vi "Double Page.vi"(8 "error in (no error)":errorcluster, 11 "Node Ptr":T1 format="%.0x") -> (0 "error out":errorcluster)   [LabVIEW 2012, in "Shared Variable Custom Device.lvlib"]
uses:
  Shared Variable Custom Device.lvlib
  <vilib>/NI Veristand/Custom Device API/Custom Device Item Ref.ctl
  <vilib>/NI Veristand/Custom Device API/Custom Device API.lvlib
panel:
  in  "Units":string
  out "Network-Published Shared Variable URL":string
  in  "Header":cluster{"Section Name":string}={"Section Name"="Custom Device Item Settings"}
  in  "Description":string
  in  "Name":string
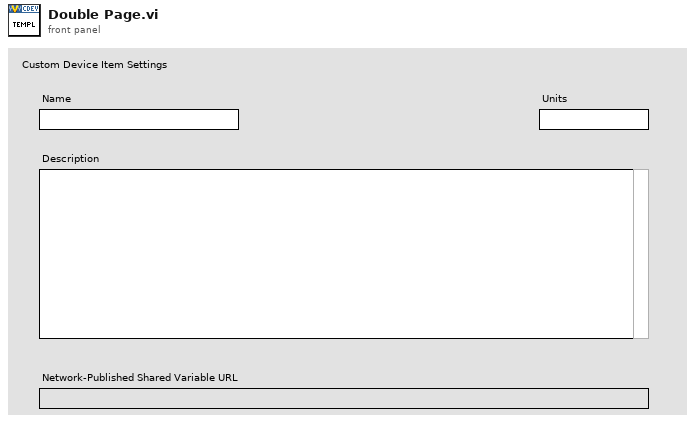
[diagram p1: front panel]
types:
  T1 = typedef "Custom Device API.lvlib/Custom Device Item Ref.ctl" = u64
  T2 = typedef "Custom Device API.lvlib/Custom Device Item Info.ctl" = cluster{"Name":string, "Is Channel":bool, "GUID":string, "Is Waveform":bool}
  T3 = typedef "Custom Device API.lvlib/Custom Device Channel.ctl" = cluster{"Type":T4, "Units":string, "Default Value":dbl, "Faultable":bool, "Scalable":bool}
  T4 = typedef "Custom Device API.lvlib/Custom Device Channel Type.ctl" = enum16{"Input", "Output"}
  T5 = typedef "Custom Device API.lvlib/Custom Device Commands.ctl" = enum16{"Default", "Item renamed", "Shutdown", "Dynamic button pressed"}
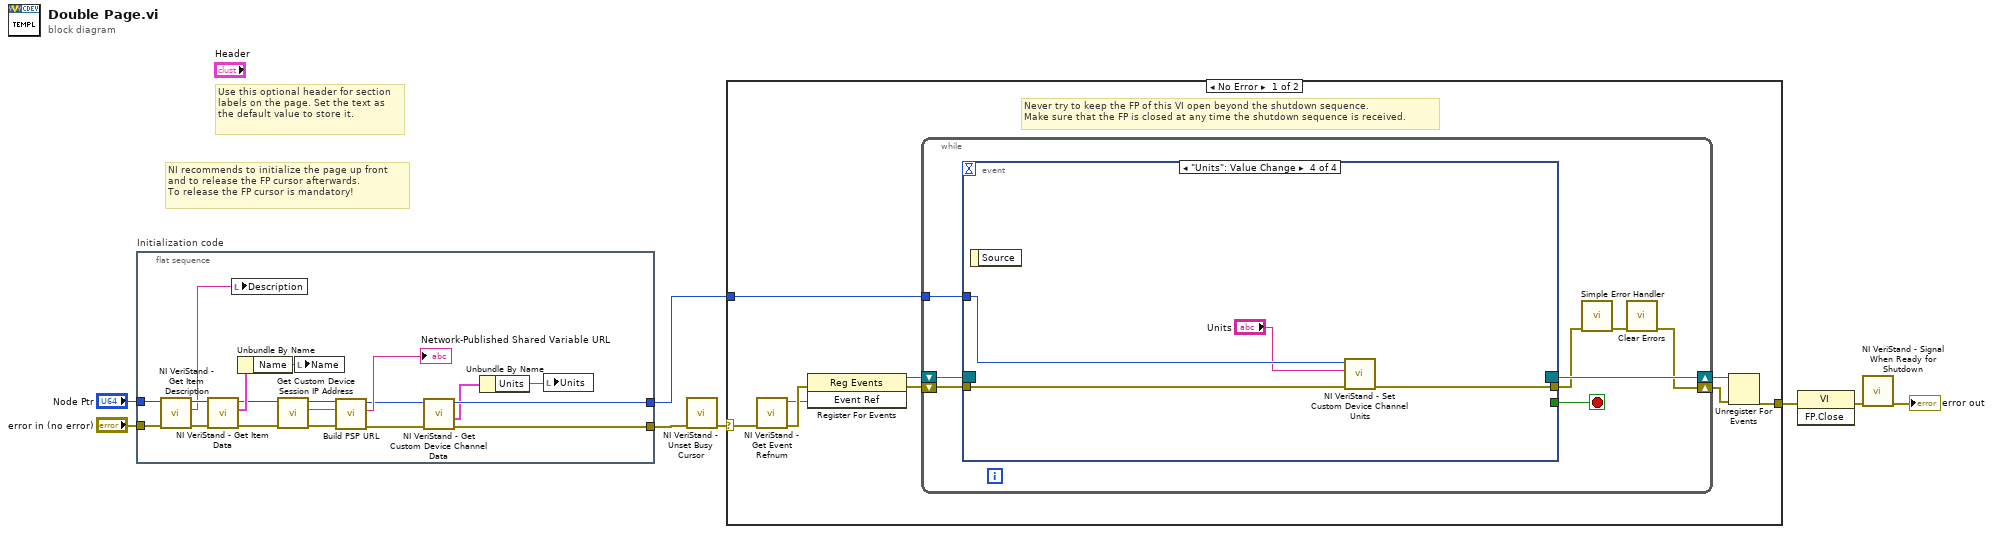
[diagram p0: block diagram]
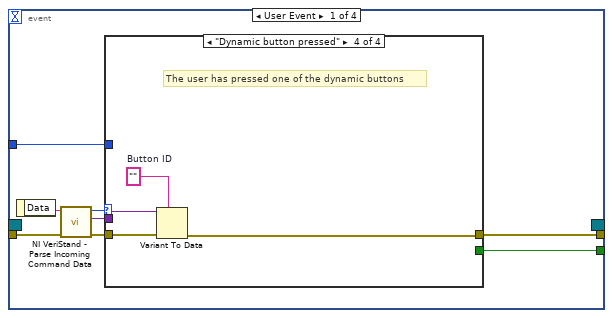
[diagram p2: hidden frame]
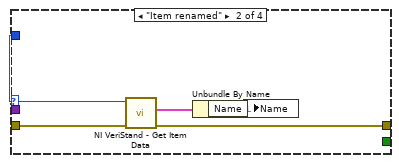
[diagram p4: hidden frame]
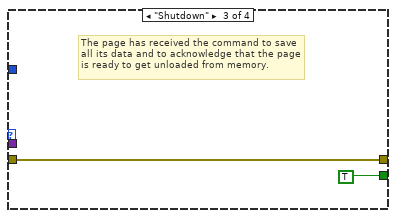
[diagram p5: hidden frame]
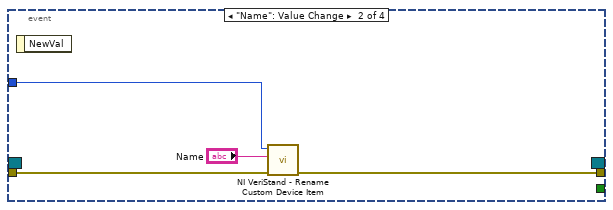
[diagram p6: hidden frame]
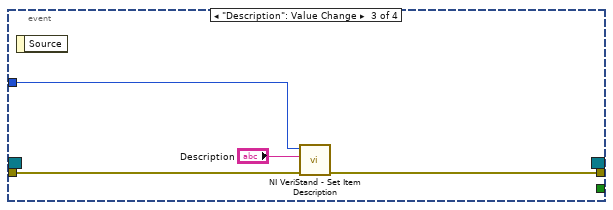
[diagram p7: hidden frame]
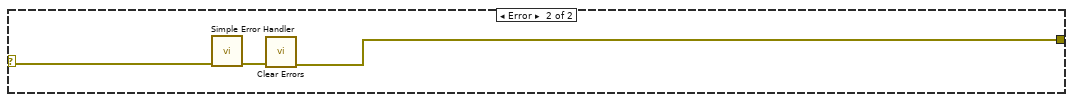
[diagram p8: hidden frame]
diagram:
  # "Use this optional header for section labels on the page. Set the text as the default value to store it."
  # "NI recommends to initialize the page up front\nand to release the FP cursor afterwards.\nTo release the FP cursor is mandatory!"
  n1 = flat-sequence "Initialization code" {
    tunnel: "error in (no error)" -> [w26]
    tunnel: "Node Ptr" -> [w25]
    tunnel: [w11] -> w4
    tunnel: [w12] -> w1
    frame #0 {
      n2 = call <vilib>:"NI VeriStand - Get Item Description.vi"("error in (no error)"=w26, "Item Ref in"=w25) -> ("error out"=w23:errorcluster, "Description"=w24:string, "Item Ref out"=w27:T1)  [unwired: 7 out]
      n3 = call <vilib>:"NI VeriStand - Get Item Data.vi"("error in (no error)"=w23, "Item Ref in"=w27) -> ("error out"=w19:errorcluster, "Item Info"=w22:T2, "Item Ref out"=w20:T1)  [unwired: 7 out]
      n4 = local write "Description"(w24) -> ()
      n5 = Unbundle By Name(w22) -> ("Name"=w21:string)
      n6 = call "Get Custom Device Session IP Address.vi"("error in (no error)"=w19, "Item Ref in"=w20) -> ("error out"=w16:errorcluster, "IP Address"=w17:string, "Item Ref out"=w18:T1)  [unwired: 7 in]
      n7 = local write "Name"(w21) -> ()
      n8 = call "Build PSP URL.vi"("error in (no error)"=w16, "IP Address"=w17, "Channel Ref in"=w18) -> ("error out"=w13:errorcluster, "Shared Variable URL"=→"Network-Published Shared Variable URL":string, "Channel Ref out"=w14:T1)  [unwired: 6 in]
      n9 = call <vilib>:"NI VeriStand - Get Custom Device Channel Data.vi"("error in (no error)"=w13, "Channel Ref in"=w14) -> ("error out"=w11:errorcluster, "Channel"=w10:T3, "Channel Ref out"=w12:T1)  [unwired: 4 in, 3 out]
      n10 = Unbundle By Name(w10) -> ("Units"=w9:string)
      n11 = local write "Units"(w9) -> ()
    }
  }
  n12 = call <vilib>:"NI VeriStand - Unset Busy Cursor.vi"("error in (no error)"=w4) -> ("error out"=w3:errorcluster)  [unwired: 10 out]
  n13 = case shown="No Error" w3 {
    selector: w3 -> [w28 w79]
    tunnel: [w33 w77] -> w8
    tunnel: w1 -> [w29 _]
    frame No Error {
      # "Never try to keep the FP of this VI open beyond the shutdown sequence.\nMake sure that the FP is closed at any time the shutdown sequence is received."
      n14 = call <vilib>:"NI VeriStand - Get Event Refnum.vi"("error in (no error)"=w28) -> ("error out"=w36:errorcluster, "Event Ref"=w32:refnum<user-event>)  [unwired: 9 out]
      n15 = register-events(error in=w36, w32) -> (reference out=w30:refnum<event-registration>, error out=w31:errorcluster)  [unwired: 1 in]
      n16 = while {
        tunnel: w29 -> [w40]
        shift-right: [w37] -> w34
        shift-left: w31 -> [w43]
        shift-right: [w44] -> w35
        shift-left: w30 -> [w42]
        stop <- w41 stop-if-true
        n17 = event shown="[3] \"Units\": Value Change" {
          selector: w42 -> [_ _ _ _]
          dyn-events: [_ _ _ _] -> w44
          timeout: _ -> [_ _ _ _]
          tunnel: w43 -> [w52 w68 w71 w75]
          tunnel: [w48 _ _ _] -> w41
          tunnel: [w47 w67 w70 w73] -> w39
          tunnel: w40 -> [w46 w66 w72 w76]
          event User Event {
            n18 = event-data() -> ("Data"=w51:string)  [unwired: 1 out]
            n19 = call <vilib>:"NI VeriStand - Parse Incoming Command Data.vi"("error in (no error)"=w52, "Incoming data"=w51) -> ("error out"=w50:errorcluster, "Outgoing data"=w45:variant, "Action"=w49:T5)  [unwired: 7 out]
            n20 = case shown="\"Dynamic button pressed\"" w49 {
              tunnel: w50 -> [w53 w58 w59 w64]
              tunnel: [_ _ TRUE _] -> w48
              tunnel: [w53 w55 w59 w61] -> w47
              tunnel: w46 -> [_ w57 _ _]
              tunnel: w45 -> [_ _ _ w63]
              frame "Default", Default {
              }
              frame "Item renamed" {
                n21 = call <vilib>:"NI VeriStand - Get Item Data.vi"("error in (no error)"=w58, "Item Ref in"=w57) -> ("error out"=w55:errorcluster, "Item Info"=w56:T2)  [unwired: 8 out]
                n22 = Unbundle By Name(w56) -> ("Name"=w54:string)
                n23 = local write "Name"(w54) -> ()
              }
              frame "Shutdown" {
                # "The page has received the command to save all its data and to acknowledge that the page is ready to get unloaded from memory."
              }
              frame "Dynamic button pressed" {
                w62 = ""  # Button ID
                # "The user has pressed one of the dynamic buttons"
                n24 = Variant To Data(error in=w64, type=w62, Variant=w63) -> (error out=w61:errorcluster)  [unwired: 1 out]
              }
            }
          }
          event "Name": Value Change {
            n25 = event-data() -> ()  [unwired: 2 out]
            n26 = call <vilib>:"NI VeriStand - Rename Custom Device Item.vi"("error in (no error)"=w68, "New Name"="Name", "Item Ref in"=w66) -> ("error out"=w67:errorcluster)  [unwired: 1 in, 7 out]
          }
          event "Description": Value Change {
            n27 = event-data() -> ()  [unwired: 2 out]
            n28 = call <vilib>:"NI VeriStand - Set Item Description.vi"("error in (no error)"=w71, "Description"="Description", "Item Ref in"=w72) -> ("error out"=w70:errorcluster)  [unwired: 8 out]
          }
          event "Units": Value Change {
            n29 = event-data() -> ()  [unwired: 2 out]
            n30 = call <vilib>:"NI VeriStand - Set Custom Device Channel Units.vi"("error in (no error)"=w75, "Units"="Units", "Channel Ref in"=w76) -> ("error out"=w73:errorcluster)  [unwired: 7 in, 1 out]
          }
        }
        n31 = call <vilib>:"Simple Error Handler.vi"("error in (no error)"=w39) -> ("error out"=w38:errorcluster)  [unwired: 1 in, 7 out]
        n32 = call <vilib>:"Clear Errors.vi"("error in (no error)"=w38) -> ("error out"=w37:errorcluster)  [unwired: 6 out]
      }
      n33 = Unregister For Events(event registration refnum=w35, error in=w34) -> (error out=w33:errorcluster)
    }
    frame Error {
      n34 = call <vilib>:"Simple Error Handler.vi"("error in (no error)"=w79) -> ("error out"=w78:errorcluster)  [unwired: 1 in, 7 out]
      n35 = call <vilib>:"Clear Errors.vi"("error in (no error)"=w78) -> ("error out"=w77:errorcluster)  [unwired: 6 out]
    }
  }
  n36 = invoke class="VI" method="FP.Close"(error in=w8) -> (error out=w7:errorcluster)  [unwired: 2 in, 2 out]
  n37 = call <vilib>:"NI VeriStand - Signal When Ready for Shutdown.vi"("error in (no error)"=w7) -> ("error out"=→"error out":errorcluster)  [unwired: 10 out]
